vi "Close.vi"(8 "error in (no error)":errorcluster, 11 "Simu Delta Robot in":refnum<class "Simu Delta Robot.lvclass">) -> (0 "error out":errorcluster, 3 "Simu Delta Robot out":refnum<class "Simu Delta Robot.lvclass">)   [LabVIEW 2013, in "Simu Delta Robot.lvclass"]
uses:
  Simu Delta Robot.lvclass
  Simu Delta Robot.lvclass/Simu Delta Robot.ctl
  <instrlib>/Hitec HS400 Series/HAIOL/Hitec HS400 Series.lvclass
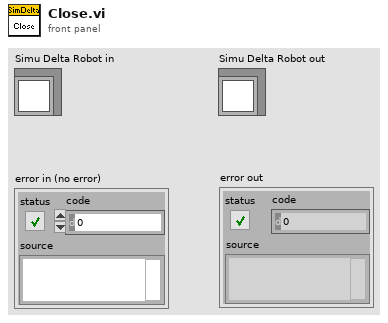
[diagram p1: front panel]
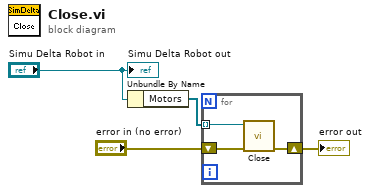
[diagram p0: block diagram]
diagram:
  n1 = Unbundle By Name("Simu Delta Robot in") -> ("Motors"=w3:refnum<class "Hitec HS400 Series.lvclass">[])
  n2 = for {
    tunnel: w3 -> [w7] mode=indexing
    shift-right: [w5] -> w1
    shift-left: "error in (no error)" -> [w6]
    n3 = call-dynamic "Close.vi"("error in (no error)"=w6, "Hitec HS400 Series in"=w7) -> ("error out"=w5:errorcluster)  [unwired: 9 in]
  }
  "error out" <- w1
  "Simu Delta Robot out" <- "Simu Delta Robot in"
